vi "Helper-GetRelativeWind.vi"(9 "Boat Angle":dbl, 10 "Current Wind":dbl) -> (2 "Relative Wind":dbl)   [LabVIEW 2013]
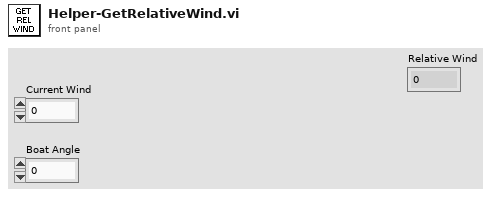
[diagram p1: front panel]
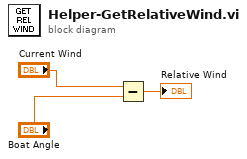
[diagram p0: block diagram]
diagram:
  n1 = Subtract(x="Current Wind", y="Boat Angle") -> (x-y=→"Relative Wind":dbl)
